vi "ARCH_AUDIT_EDITOR_click_discard.vi"(10 "CellPosition":T2, 11 "event_structure_shift_register_in":T1={"REF_EDIT_clicked_row"=-1, "REF_EDIT_selected_row"=-1, "SQL_EDIT_clicked_row"=-1, "SQL_EDIT_selected_row"=-1, "ARCH_EDIT_selected_row"=-1, "ARCH_EDIT_clicked_row"=-1, "ARCH_AUDIT_EDIT_selected_row"=-1, "ARCH_AUDIT_EDIT_clicked_row"=-1, "USER_EDIT_selected_row"=-1, "USER_EDIT_clicked_row"=-1, "REPORT_GEAR_toggle_all_results"=FALSE, "REPORT_AUDIT_toggle_all_results"=FALSE}) -> (2 "Discard?":bool, 3 "event_structure_shift_register_out":T1={"REF_EDIT_clicked_row"=-1, "REF_EDIT_selected_row"=-1, "SQL_EDIT_clicked_row"=-1, "SQL_EDIT_selected_row"=-1, "ARCH_EDIT_selected_row"=-1, "ARCH_EDIT_clicked_row"=-1, "ARCH_AUDIT_EDIT_selected_row"=-1, "ARCH_AUDIT_EDIT_clicked_row"=-1, "USER_EDIT_selected_row"=-1, "USER_EDIT_clicked_row"=-1, "REPORT_GEAR_toggle_all_results"=FALSE, "REPORT_AUDIT_toggle_all_results"=FALSE})   [LabVIEW 2020]
uses:
  CLIENT_event_structure_shift_register.ctl
  <vilib>/Utility/miscctls.llb/LVRowAndColumnTypeDef.ctl
  FGV/ARCH_AUDIT_EDITOR_records_display/FGV_ARCH_AUDIT_EDITOR_records_display.ctl
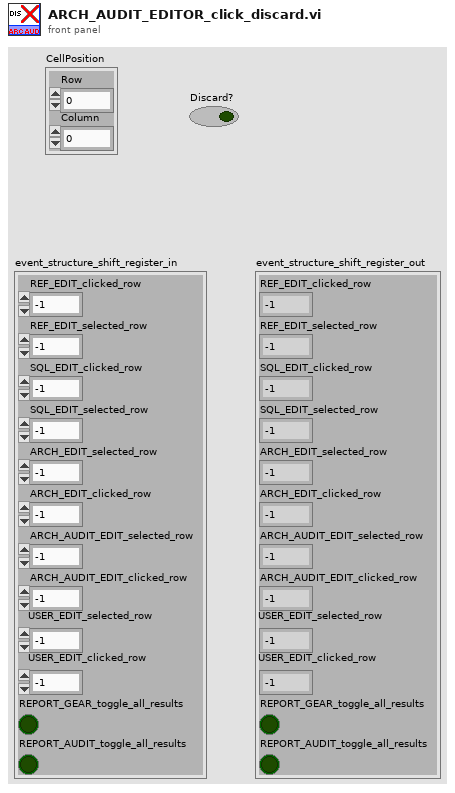
[diagram p1: front panel]
types:
  T1 = typedef "CLIENT_event_structure_shift_register.ctl" = cluster{"REF_EDIT_clicked_row":i32, "REF_EDIT_selected_row":i32, "SQL_EDIT_clicked_row":i32, "SQL_EDIT_selected_row":i32, "ARCH_EDIT_selected_row":i32, "ARCH_EDIT_clicked_row":i32, "ARCH_AUDIT_EDIT_selected_row":i32, "ARCH_AUDIT_EDIT_clicked_row":i32, "USER_EDIT_selected_row":i32, "USER_EDIT_clicked_row":i32, "REPORT_GEAR_toggle_all_results":bool, "REPORT_AUDIT_toggle_all_results":bool}
  T2 = typedef "LVRowAndColumnTypeDef.ctl" = cluster{"Row":i32, "Column":i32}
  T3 = typedef "FGV_ARCH_AUDIT_EDITOR_records_display.ctl" = enum16{"initialize", "set_arch_cfg_tables_names", "set_station_number", "set_type_filter", "set_headers", "set_records", "get_arch_cfg_table_name", "get_arch_cfg_hist_table_name", "get_station_number", "get_type_filter", "get_headers", "get_uneditable_columns", "get_all_info", "record_added?", "record_inserted?", "record_edited?", "record_updated?", "record_deleted?", "discard_changes"}
  T4 = typedef "ARCH_AUDIT_EDITOR_all_info.ctl" = cluster{"station_number":string, "type_filter":string, "archivisation_audit_cfg_table":string, "archivisation_audit_cfg_history":string, "column_names":string[], "uneditable_columns":string[], "uneditable_columns":i32[], "editable_columns":i32[], "values_in_database":string[][], "size":cluster{"columns":i32, "SQL_rows":i32, "disp_rows":i32}, "ARCH_AUDIT_record_states":T5[]}
  T5 = typedef "SQL_record_states.ctl" = enum16{"Equal", "Added", "Edited", "Deleted"}
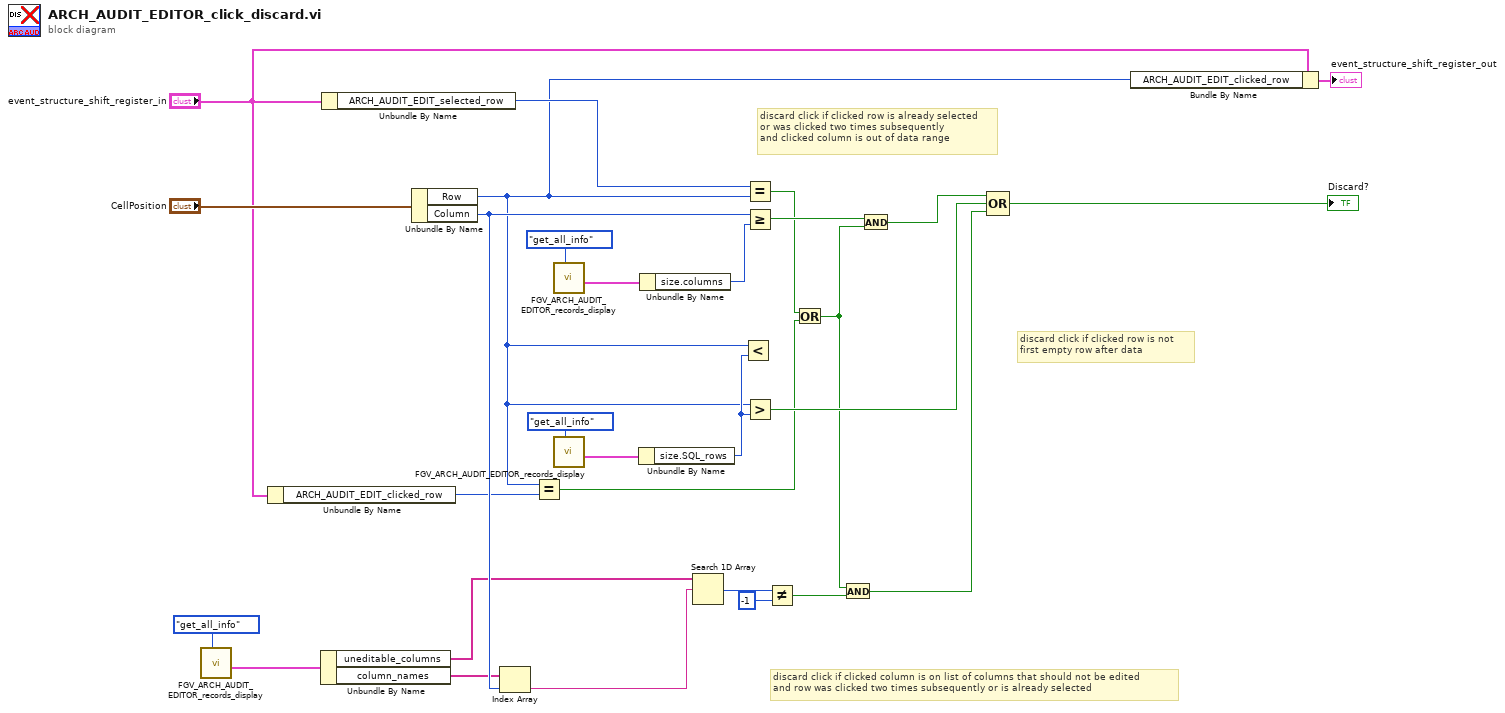
[diagram p0: block diagram]
diagram:
  # "discard click if clicked column is on list of columns that should not be edited\nand row was clicked two times subsequently or is already selected"
  # "discard click if clicked row is not \nfirst empty row after data"
  # "discard click if clicked row is already selected\nor was clicked two times subsequently\nand clicked column is out of data range"
  n1 = call "FGV_ARCH_AUDIT_EDITOR_records_display.vi"("options"=FGV_ARCH_AUDIT_EDITOR_records_display."get_all_info") -> ("all_info"=w5:T4)  [unwired: 7 in, 3 out]
  n2 = Unbundle By Name("event_structure_shift_register_in") -> ("ARCH_AUDIT_EDIT_clicked_row"=w15:i32)
  n3 = Unbundle By Name(w5) -> ("uneditable_columns"=w8:string[], "column_names"=w9:string[])
  n4 = Unbundle By Name("event_structure_shift_register_in") -> ("ARCH_AUDIT_EDIT_selected_row"=w19:i32)
  n5 = Unbundle By Name("CellPosition") -> ("Row"=w14:i32, "Column"=w27:i32)
  n6 = Index Array(array=w9, index=w27) -> (element=w26:string)
  n7 = Equal?(x=w14, y=w15) -> (x = y?=w11:bool)
  n8 = call "FGV_ARCH_AUDIT_EDITOR_records_display.vi"("options"=FGV_ARCH_AUDIT_EDITOR_records_display."get_all_info") -> ("all_info"=w1:T4)  [unwired: 7 in, 3 out]
  n9 = call "FGV_ARCH_AUDIT_EDITOR_records_display.vi"("options"=FGV_ARCH_AUDIT_EDITOR_records_display."get_all_info") -> ("all_info"=w3:T4)  [unwired: 7 in, 3 out]
  n10 = Unbundle By Name(w3) -> ("size.SQL_rows"=w18:i32)
  n11 = Unbundle By Name(w1) -> ("size.columns"=w29:i32)
  n12 = Search 1D Array(1D array=w8, element=w26) -> (index of element=w25:i32)  [unwired: 1 in]
  n13 = Less?(x=w14, y=w18) -> ()  [unwired: 1 out]
  n14 = Equal?(x=w19, y=w14) -> (x = y?=w12:bool)
  n15 = Greater Or Equal?(x=w27, y=w29) -> (x >= y?=w13:bool)
  n16 = Greater?(x=w14, y=w18) -> (0:w20:bool)
  n17 = Not Equal?(x=w25, y=-1) -> (x != y?=w17:bool)
  n18 = Or(x=w12, y=w11) -> (x .or. y?=w10:bool)
  n19 = And(x=w10, y=w17) -> (x .and. y?=w22:bool)
  n20 = And(x=w13, y=w10) -> (x .and. y?=w23:bool)
  n21 = Compound Arithmetic op=OR(w23, w20, w22) -> (→"Discard?":bool)
  n22 = Bundle By Name(cluster="event_structure_shift_register_in", "ARCH_AUDIT_EDIT_clicked_row"=w14) -> (→"event_structure_shift_register_out":T1)
